vi "Set grpc_reflection_v1alpha_ServerReflectionResponse.vi"(7 "Complete Call (T)":bool=TRUE, 8 "error in (no error)":errorcluster, 10 "package_templatemessage":T1, 11 "gRPCid":T3) -> (0 "error out":errorcluster)   [LabVIEW 2025, in "reflection_server.lvlib"]
uses:
  reflection_server.lvlib
  <vilib>/gRPC/LabVIEW gRPC Library/Shared/grpcId.ctl
  grpc_reflection_v1alpha_ServerReflectionResponse.ctl
  grpc_reflection_v1alpha_ServerReflectionRequest_message_request/grpc_reflection_v1alpha_ServerReflectionRequest_message_request.lvclass
  grpc_reflection_v1alpha_ServerReflectionResponse_message_response/grpc_reflection_v1alpha_ServerReflectionResponse_message_response.lvclass
  grpc_reflection_v1alpha_ServerReflectionRequest.ctl
  grpc_reflection_v1alpha_ServerReflectionResponse_Flat.ctl
  grpc_reflection_v1alpha_ServerReflectionRequest_Flat.ctl
  grpc_reflection_v1alpha_ExtensionRequest_Flat.ctl
  grpc_reflection_v1alpha_FileDescriptorResponse_Flat.ctl
  grpc_reflection_v1alpha_ExtensionNumberResponse_Flat.ctl
  grpc_reflection_v1alpha_ListServiceResponse_Flat.ctl
  grpc_reflection_v1alpha_ServiceResponse_Flat.ctl
  grpc_reflection_v1alpha_ErrorResponse_Flat.ctl
  grpc_reflection_v1alpha_ServerReflectionRequest_message_request/grpc_reflection_v1alpha_ServerReflectionRequest_message_request.lvclass/grpc_reflection_v1alpha_ServerReflectionRequest_message_request.ctl
  grpc_reflection_v1alpha_ServerReflectionResponse_message_response/grpc_reflection_v1alpha_ServerReflectionResponse_message_response.lvclass/grpc_reflection_v1alpha_ServerReflectionResponse_message_response.ctl
  dcc74a39-081a-4bdd-860b-8ed792803c96.vi
  RichToFlatgrpc_reflection_v1alpha_ServerReflectionRequest.vi
  grpc_reflection_v1alpha_ServerReflectionResponse_message_response/GetActiveFieldIndex.vi
  grpc_reflection_v1alpha_ServerReflectionResponse_message_response/Getfile_descriptor_response.vi
  RichToFlatgrpc_reflection_v1alpha_FileDescriptorResponse.vi
  grpc_reflection_v1alpha_ServerReflectionResponse_message_response/Getall_extension_numbers_response.vi
  RichToFlatgrpc_reflection_v1alpha_ExtensionNumberResponse.vi
  grpc_reflection_v1alpha_ServerReflectionResponse_message_response/Getlist_services_response.vi
  RichToFlatgrpc_reflection_v1alpha_ListServiceResponse.vi
  grpc_reflection_v1alpha_ServerReflectionResponse_message_response/Geterror_response.vi
  RichToFlatgrpc_reflection_v1alpha_ErrorResponse.vi
  <vilib>/gRPC/LabVIEW gRPC Library/Shared/TranslateGrpcError.vi
  grpc_reflection_v1alpha_ServerReflectionRequest_message_request/GetActiveFieldIndex.vi
  grpc_reflection_v1alpha_ServerReflectionRequest_message_request/Getfile_by_filename.vi
  grpc_reflection_v1alpha_ServerReflectionRequest_message_request/Getfile_containing_symbol.vi
  grpc_reflection_v1alpha_ServerReflectionRequest_message_request/Getfile_containing_extension.vi
  RichToFlatgrpc_reflection_v1alpha_ExtensionRequest.vi
  grpc_reflection_v1alpha_ServerReflectionRequest_message_request/Getall_extension_numbers_of_type.vi
  grpc_reflection_v1alpha_ServerReflectionRequest_message_request/Getlist_services.vi
  RichToFlatgrpc_reflection_v1alpha_ServiceResponse.vi
  <vilib>/gRPC/LabVIEW gRPC Library/Server API/Server/Get Server DLL Path.vi
  <vilib>/Utility/error.llb/Error Cluster From Error Code.vi
  <vilib>/gRPC/LabVIEW gRPC Library/grpc-lvsupport-release.lvlib
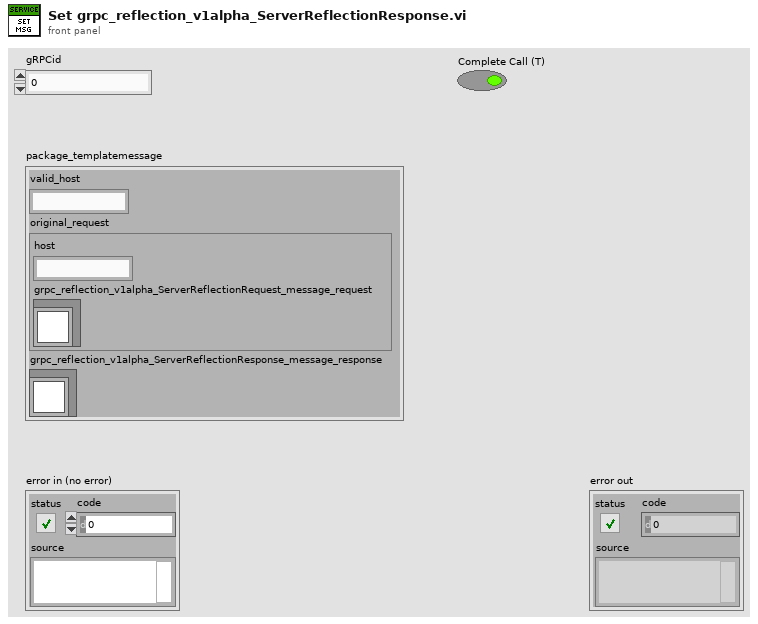
[diagram p1: front panel]
types:
  T1 = typedef "reflection_server.lvlib/grpc_reflection_v1alpha_ServerReflectionResponse.ctl" = cluster{"valid_host":string, "original_request":T2, "grpc_reflection_v1alpha_ServerReflectionResponse_message_response":refnum<class "grpc_reflection_v1alpha_ServerReflectionResponse_message_response.lvclass">}
  T2 = typedef "reflection_server.lvlib/grpc_reflection_v1alpha_ServerReflectionRequest.ctl" = cluster{"host":string, "grpc_reflection_v1alpha_ServerReflectionRequest_message_request":refnum<class "grpc_reflection_v1alpha_ServerReflectionRequest_message_request.lvclass">}
  T3 = typedef "grpc-lvsupport-release.lvlib/grpcId.ctl" = u64
  T4 = typedef "reflection_server.lvlib/grpc_reflection_v1alpha_ServerReflectionResponse_Flat.ctl" = cluster{"valid_host":string, "original_request":T5, "grpc_reflection_v1alpha_ServerReflectionResponse_message_response_selected_index":i32, "file_descriptor_response":T7, "all_extension_numbers_response":T8, "list_services_response":T9, "error_response":T11}
  T5 = typedef "reflection_server.lvlib/grpc_reflection_v1alpha_ServerReflectionRequest_Flat.ctl" = cluster{"host":string, "grpc_reflection_v1alpha_ServerReflectionRequest_message_request_selected_index":i32, "file_by_filename":string, "file_containing_symbol":string, "file_containing_extension":T6, "all_extension_numbers_of_type":string, "list_services":string}
  T6 = typedef "reflection_server.lvlib/grpc_reflection_v1alpha_ExtensionRequest_Flat.ctl" = cluster{"containing_type":string, "extension_number":i32}
  T7 = typedef "reflection_server.lvlib/grpc_reflection_v1alpha_FileDescriptorResponse_Flat.ctl" = cluster{"file_descriptor_proto":cluster{"Array":u8[]}[]}
  T8 = typedef "reflection_server.lvlib/grpc_reflection_v1alpha_ExtensionNumberResponse_Flat.ctl" = cluster{"base_type_name":string, "extension_number":i32[]}
  T9 = typedef "reflection_server.lvlib/grpc_reflection_v1alpha_ListServiceResponse_Flat.ctl" = cluster{"service":T10[]}
  T10 = typedef "reflection_server.lvlib/grpc_reflection_v1alpha_ServiceResponse_Flat.ctl" = cluster{"name":string}
  T11 = typedef "reflection_server.lvlib/grpc_reflection_v1alpha_ErrorResponse_Flat.ctl" = cluster{"error_code":i32, "error_message":string}
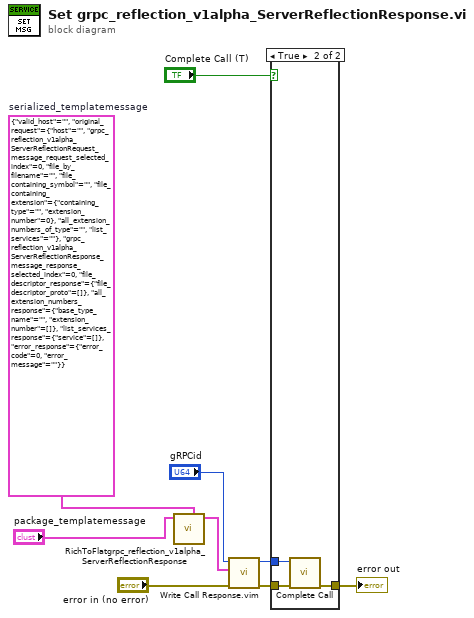
[diagram p0: block diagram]
diagram:
  w2 = T4 {"valid_host"="", "original_request"={"host"="", "grpc_reflection_v1alpha_ServerReflectionRequest_message_request_selected_index"=0, "file_by_filename"="", "file_containing_symbol"="", "file_containing_extension"={"containing_type"="", "extension_number"=0}, "all_extension_numbers_of_type"="", "list_services"=""}, "grpc_reflection_v1alpha_ServerReflectionResponse_message_response_selected_index"=0, "file_descriptor_response"={"file_descriptor_proto"=[]}, "all_extension_numbers_response"={"base_type_name"="", "extension_number"=[]}, "list_services_response"={"service"=[]}, "error_response"={"error_code"=0, "error_message"=""}}  # serialized_templatemessage
  n1 = call "RichToFlatgrpc_reflection_v1alpha_ServerReflectionResponse.vi"("OutputClusterType"=w2, "InputCluster"="package_templatemessage") -> ("OutputCluster"=w1:T4)  [unwired: 9 in]
  n2 = call "Write Call Response.vim"("error in"="error in (no error)", "Response Data"=w1, "gRPCid in"="gRPCid") -> ("error out"=w6:errorcluster, "gRPCid out"=w7:T3)  [unwired: 7 in]
  n3 = case shown="True" "Complete Call (T)" {
    tunnel: [w10 w13] -> w9
    tunnel: w7 -> [_ w12]
    tunnel: w6 -> [w10 w11]
    frame False {
    }
    frame True {
      n4 = call <vilib>:"Complete Call.vi"("gRPCid"=w12, "error in"=w11) -> ("error out"=w13:errorcluster)  [unwired: 8 in]
    }
  }
  "error out" <- w9
